vi "SubCycles list.vi"() -> (1 "Canceled":bool, 2 "Subcycle name":string)   [LabVIEW 2014]
panel:
  in  "Cancel Button":bool
  in  "OK Button":bool
  in  "Subcycle List":i32(listbox)=2
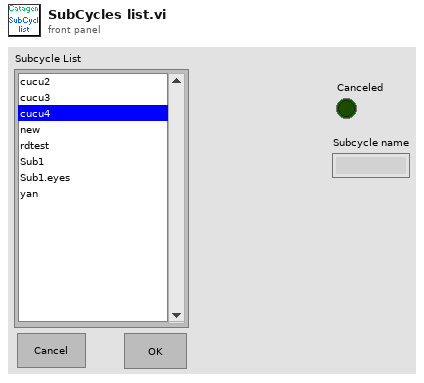
[diagram p1: front panel]
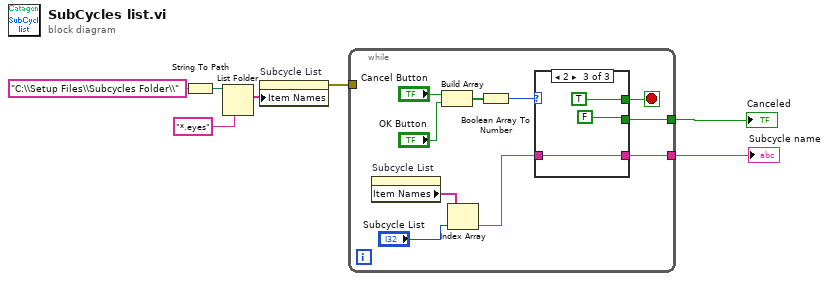
[diagram p0: block diagram]
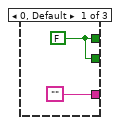
[diagram p2: hidden frame]
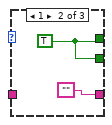
[diagram p3: hidden frame]
diagram:
  n1 = String To Path(string="C:\\Setup Files\\Subcycles Folder\\") -> (path=w5:path)
  n2 = List Folder(path=w5, pattern="*.eyes") -> (filenames=w3:string[])  [unwired: 2 in, 3 out]
  n3 = property on="Subcycle List" class="LstBox (strict)"("Item Names"=w3) -> (error out=w2:errorcluster)  [unwired: 2 in, 1 out]
  n4 = while {
    tunnel: [w12] -> w7
    tunnel: [w11] -> w6
    tunnel: w2 -> [_]
    stop <- w13 stop-if-true
    n5 = property on="Subcycle List" class="LstBox (strict)"() -> ("Item Names"=w10:string[])  [unwired: 2 in, 2 out]
    n6 = Build Array("Cancel Button", "OK Button") -> (w15:bool[])
    n7 = Index Array(array=w10, index="Subcycle List") -> (element=w8:string)
    n8 = Boolean Array To Number(Boolean array=w15) -> (number=w14:u32)
    n9 = case shown="2" w14 {
      tunnel: w8 -> [_ _ w22]
      tunnel: [w18 w21 TRUE] -> w13
      tunnel: [w18 w21 FALSE] -> w12
      tunnel: ["" "" w22] -> w11
      frame 0, Default {
        w18 = FALSE
      }
      frame 1 {
        w21 = TRUE
      }
      frame 2 {
      }
    }
  }
  "Subcycle name" <- w6
  "Canceled" <- w7
